vi "Scale_Plot.vi"(0 "Cluster":cluster{"Y":dbl[], "X":dbl[]}, 2 "String":string) -> (5 "Cluster 2":cluster{"Y":dbl[], "X":dbl[]})   [LabVIEW 2019]
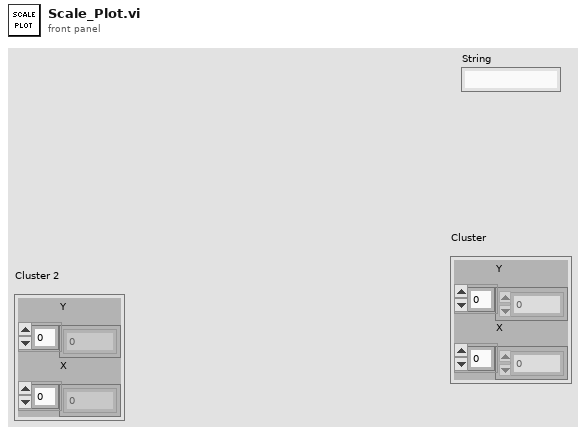
[diagram p1: front panel]
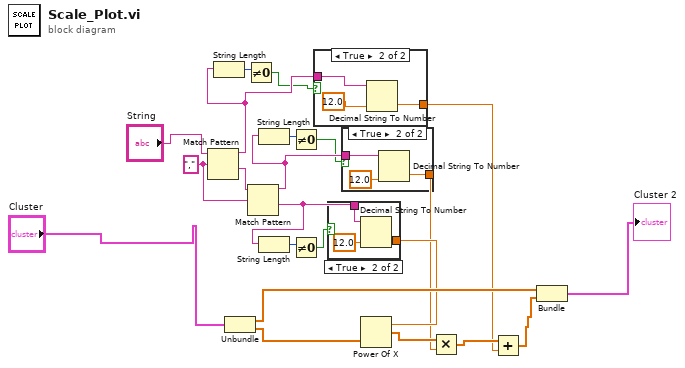
[diagram p0: block diagram]
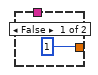
[diagram p2: hidden frame]
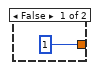
[diagram p3: hidden frame]
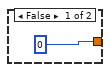
[diagram p4: hidden frame]
diagram:
  w15 = "," ("regular expression")
  n1 = Match Pattern(string="String", regular expression=w15) -> (before substring=w3:string, after substring=w16:string)  [unwired: 1 in, 2 out]
  n2 = String Length(string=w3) -> (length=w4:i32)
  n3 = Unbundle("Cluster") -> ("Y"=w21:dbl[], "X"=w20:dbl[])
  n4 = Not Equal To 0?(x=w4) -> (x != 0?=w2:bool)
  n5 = Match Pattern(string=w16, regular expression=w15) -> (before substring=w6:string, after substring=w8:string)  [unwired: 1 in, 2 out]
  n6 = String Length(string=w6) -> (length=w7:i32)
  n7 = String Length(string=w8) -> (length=w10:i32)
  n8 = Not Equal To 0?(x=w7) -> (x != 0?=w5:bool)
  n9 = Not Equal To 0?(x=w10) -> (x != 0?=w9:bool)
  n10 = case shown="True" w2 {
    tunnel: [0 w26] -> w11
    tunnel: w3 -> [_ w25]
    frame False {
    }
    frame True {
      n11 = Decimal String To Number(string=w25, default (0L)=12.0) -> (number=w26:dbl)  [unwired: 1 in, 1 out]
    }
  }
  n12 = case shown="True" w9 {
    tunnel: [1 w30] -> w19
    tunnel: w8 -> [_ w29]
    frame False {
    }
    frame True {
      n13 = Decimal String To Number(string=w29, default (0L)=12.0) -> (number=w30:dbl)  [unwired: 1 in, 1 out]
    }
  }
  n14 = case shown="True" w5 {
    tunnel: w6 -> [_ w34]
    tunnel: [1 w33] -> w13
    frame False {
    }
    frame True {
      n15 = Decimal String To Number(string=w34, default (0L)=12.0) -> (number=w33:dbl)  [unwired: 1 in, 1 out]
    }
  }
  n16 = Power Of X(1:w20, 2:w19) -> (0:w14:dbl[])
  n17 = Multiply(x=w14, y=w13) -> (x*y=w12:dbl[])
  n18 = Add(x=w12, y=w11) -> (x+y=w1:dbl[])
  n19 = Bundle("Y"=w21, w1) -> (→"Cluster 2":cluster{"Y":dbl[], dbl[]})  [unwired: 1 in]
